vi "Measurement.WavelengthSweeping.UI.GetDependencies.vi"(8 "error in (no error)":errorcluster, 11 "Measurement.WavelengthSweeping.UI in":refnum<class "Measurement.WavelengthSweeping.UI.lvclass">) -> (0 "error out":errorcluster, 2 "Dependencies":T1, 3 "Measurement.WavelengthSweeping.UI out":refnum<class "Measurement.WavelengthSweeping.UI.lvclass">)   [LabVIEW 2017, in "Measurement.WavelengthSweeping.UI.lvclass"]
uses:
  Measurement.WavelengthSweeping.UI.lvclass
  Typedefs/Dependencies--Cluster.ctl
  Measurement.WavelengthSweeping/Measurement.WavelengthSweeping.lvclass
  Measurement.WavelengthSweeping.UI.lvclass/Measurement.WavelengthSweeping.UI.ctl
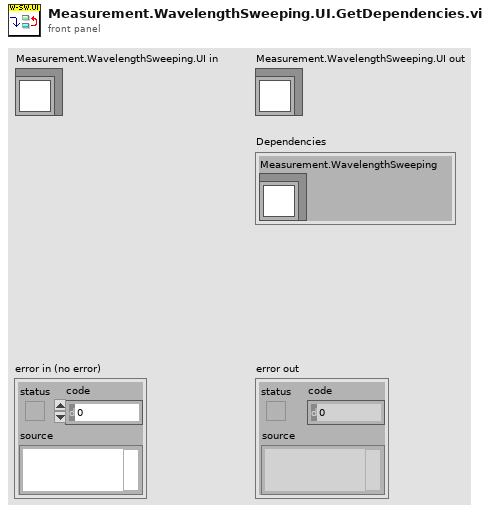
[diagram p1: front panel]
types:
  T1 = typedef "Measurement.WavelengthSweeping.UI.lvclass/Dependencies--Cluster.ctl" = cluster{"Measurement.WavelengthSweeping":refnum<class "Measurement.WavelengthSweeping.lvclass">}
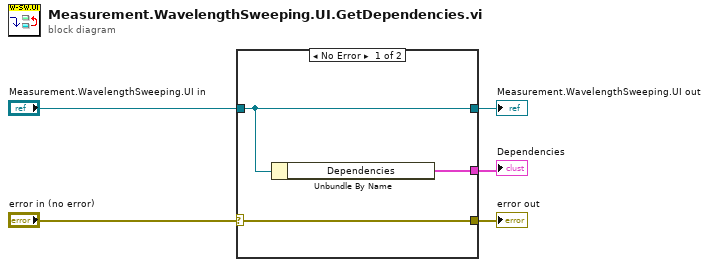
[diagram p0: block diagram]
diagram:
  n1 = case shown="No Error" "error in (no error)" {
    selector: "error in (no error)" -> [w8 w10]
    tunnel: [w8 w10] -> w4
    tunnel: [w7 w9] -> w2
    tunnel: "Measurement.WavelengthSweeping.UI in" -> [w7 w9]
    tunnel: [w6 _] -> w1
    frame No Error {
      n2 = Unbundle By Name(w7) -> ("Dependencies"=w6:T1)
    }
    frame Error {
    }
  }
  "error out" <- w4
  "Measurement.WavelengthSweeping.UI out" <- w2
  "Dependencies" <- w1
